vi "UI_DetachFrom_Subpanel.vi"(8 "error in (no error)":errorcluster, 10 "Sub Panel":refnum<vi>, 11 "UI_Actor in":refnum<class "UI_Actor.lvclass">) -> (0 "error out":errorcluster, 3 "UI_Actor out":refnum<class "UI_Actor.lvclass">)   [LabVIEW 2015]
uses:
  UI_Actor.lvclass
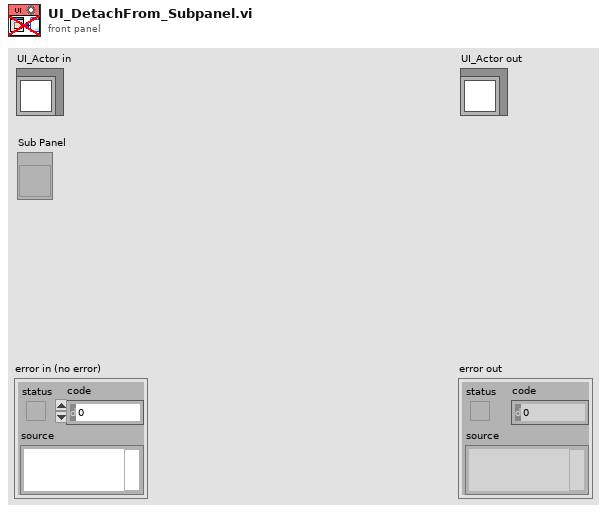
[diagram p1: front panel]
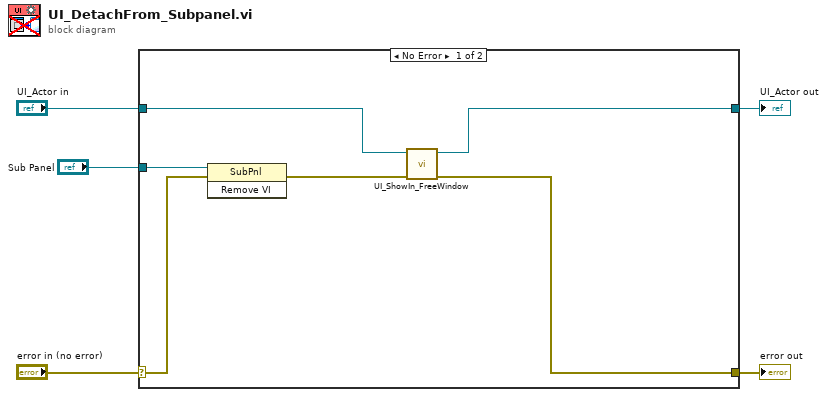
[diagram p0: block diagram]
diagram:
  n1 = case shown="No Error" "error in (no error)" {
    selector: "error in (no error)" -> [w9 w13]
    tunnel: [w8 w13] -> w4
    tunnel: [w6 w12] -> w2
    tunnel: "UI_Actor in" -> [w7 w12]
    tunnel: "Sub Panel" -> [w11 _]
    frame No Error {
      n2 = invoke on="Invoke Node" class="SubPnl" method="Remove VI"(reference=w11, error in=w9) -> (error out=w10:errorcluster)  [unwired: 1 in, 2 out]
      n3 = call-dynamic "UI_ShowIn_FreeWindow.vi"("error in (no error)"=w10, "UI_Actor in"=w7) -> ("error out"=w8:errorcluster, "UI_Actor out"=w6:refnum<class "UI_Actor.lvclass">)  [unwired: 8 in]
    }
    frame Error {
    }
  }
  "error out" <- w4
  "UI_Actor out" <- w2
